vi "Insight_Telnet_Laser_Close-Session.vi"(8 "error in (no error)":errorcluster, 11 "telnet connection":T1) -> (0 "error out":errorcluster, 1 "response data":string, 3 "telnet  connection out":T1)   [LabVIEW 2011]
doc: "Insight Photonic Solutions\n\nThis VI commands the Telnet session to close within the laser. Afterwards, close the PC's Telnet Session using \"Insight_Telnet_Proper-Close.vi\".\n\nver 1.0 - original release"
uses:
  Telnet Session.ctl
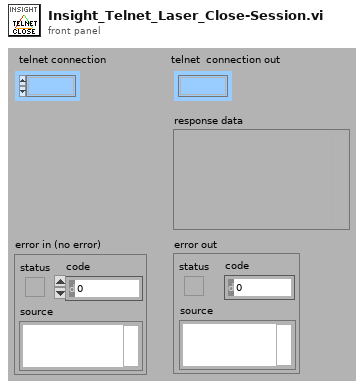
[diagram p1: front panel]
types:
  T1 = typedef "Telnet Session.ctl" = refnum<k1>
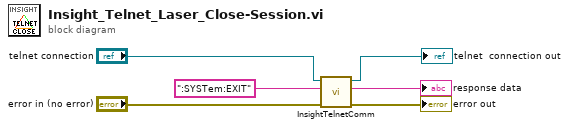
[diagram p0: block diagram]
diagram:
  n1 = call "InsightTelnetComm.vi"("error in"="error in (no error)", "write buffer (\"\")"=":SYSTem:EXIT" ("String"), "telnet connection"="telnet connection") -> ("error out"=→"error out":errorcluster, "response data"=→"response data":string, "telnet  connection out"=→"telnet  connection out":T1)  [unwired: 4 in]
